vi "CreateIntegerArray.vi"(1 "Int Array":T1={"Minimum"=10, "Maximum"=10000, "# of Points"=1999, "Spacing"=enum."Linear"}) -> (0 "Array":i32[](array[numeric]))   [LabVIEW 2015]
uses:
  <vilib>/imath/engines/lvmath2/RunTimeEngine/Managers/WorkSpace/UID Generator.vi
  <vilib>/imath/engines/lvmath2/RunTimeEngine/RunTimeType/NIMS_RunTimeType_From StrictType (excl LVString).vi
  <instcachedir>/0/NIMS_RunTimeType_From StrictType (excl LVString)_EB1C38A9BC5048DA9ABDA8F781E54D21.lvgen/NIMS_RunTimeType_From StrictType (excl LVString)_EB1C38A9BC5048DA9ABDA8F781E54D21_000.vi
  <vilib>/imath/engines/lvmath2/RunTimeEngine/LocalVariableDefStatement/MC_LocalVariableDefStatement_Display.vi
  <vilib>/imath/engines/lvmath2/RunTimeSupport/NIMS_Complex To Real.vi
  <instcachedir>/0/NIMS_Complex To Real_01315F44AA8B4CE79FEF95AE999DC25E.lvgen/NIMS_Complex To Real_01315F44AA8B4CE79FEF95AE999DC25E_001.vi
  <vilib>/imath/engines/lvmath2/RunTimeEngine/BuiltInFunctions/logramp/NIMS_logramp.vi
  <vilib>/imath/engines/lvmath2/RunTimeEngine/ErrorHandling/NIMS_Create Error From Enums.vi
  <vilib>/imath/engines/lvmath2/RunTimeEngine/BuiltInFunctions/linramp/NIMS_linramp.vi
  <vilib>/imath/engines/lvmath2/RunTimeEngine/Managers/SymbolTable/Clear UID.vi
  <vilib>/imath/engines/lvmath2/RunTimeEngine/NodeEndStatement/NIMS_NodeEndStatement_Output.vi
  <instcachedir>/0/NIMS_NodeEndStatement_Output_53EC0D466D134D7ABD903AC30B43404B.lvgen/NIMS_NodeEndStatement_Output_53EC0D466D134D7ABD903AC30B43404B_004.vi
  <vilib>/imath/engines/lvmath2/RunTimeEngine/ErrorHandling/NIMS_Finalize Error.vi
  <vilib>/imath/engines/lvmath2/RunTimeEngine/Managers/SymbolTable/NIMS_WorkSpace.lvlib
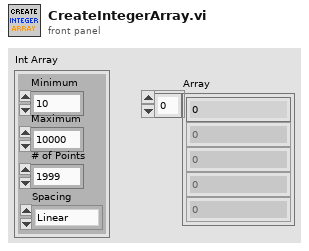
[diagram p1: front panel]
types:
  T1 = cluster{"Minimum":i32, "Maximum":i32, "# of Points":i32, "Spacing":enum16{"Linear", "Logarithmic"}}
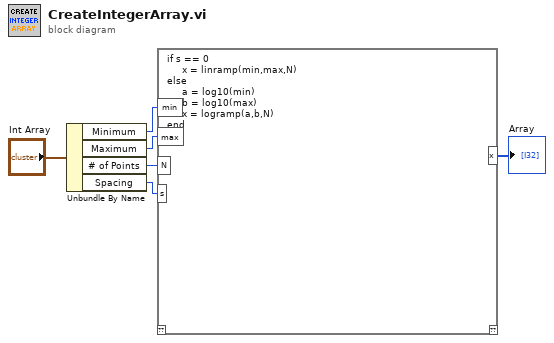
[diagram p0: block diagram]
diagram:
  n1 = Unbundle By Name("Int Array") -> ("Minimum"=w4:i32, "Maximum"=w3:i32, "# of Points"=w2:i32, "Spacing"=w1:enum16{"Linear", "Logarithmic"})
  n2 = mathscript code="if s == 0\n     x = linramp(min,max,N)\nelse\n     a = log10(min)\n     b = log10(max)\n     x = logramp(a,b,N)\nend"("min"=w4, "max"=w3, "s"=w1, "N"=w2) -> ("x"=→"Array":i32[])  [unwired: 1 in, 1 out]
